vi "decade.vi"(0 "Data In":T5, 2 "Display State In":T3, 3 "Container State":T4) -> (6 "Data Out":T5, 7 "Display State Out":T3, 8 "Action":T2)   [LabVIEW 2017, in "XGaussfitGraph.lvlib" / "XGaussfitGraph.xctl"]
uses:
  XGaussfitGraph.xctl
  Data.ctl
  <vilib>/_xctls/Container State.ctl
  State.ctl
  <vilib>/_xctls/Action.ctl
  Support/Def-UI-Properties.ctl
  <vilib>/_xctls/XControlSupport.lvlib
panel:
  out "Props":T1
  out "Data":dbl[][](graph)
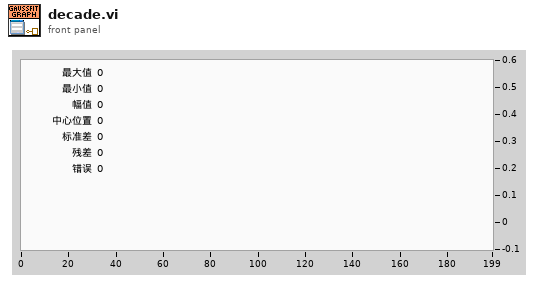
[diagram p1: front panel]
types:
  T1 = typedef "XGaussfitGraph.lvlib/XGaussfitGraph.xctl/Def-UI-Properties.ctl" = cluster{"max value":dbl, "min value":dbl, "amplitude":dbl, "center":dbl, "deviation":dbl, "residue":dbl, "error":i32}
  T2 = typedef "XControlSupport.lvlib/Action.ctl" = cluster{"Data Changed?":bool, "State Changed?":bool, "Action Name":string}
  T3 = typedef "XGaussfitGraph.lvlib/XGaussfitGraph.xctl/State.ctl" = cluster{"Numeric":dbl, "Y.scale":cluster{"auto?":bool, "max":dbl, "min":dbl}}
  T4 = typedef "XControlSupport.lvlib/Container State.ctl" = cluster{"Indicator?":bool, "Run Mode?":bool, " Refnum":refnum<vi>}
  T5 = typedef "XGaussfitGraph.lvlib/XGaussfitGraph.xctl/Data.ctl" = dbl[]
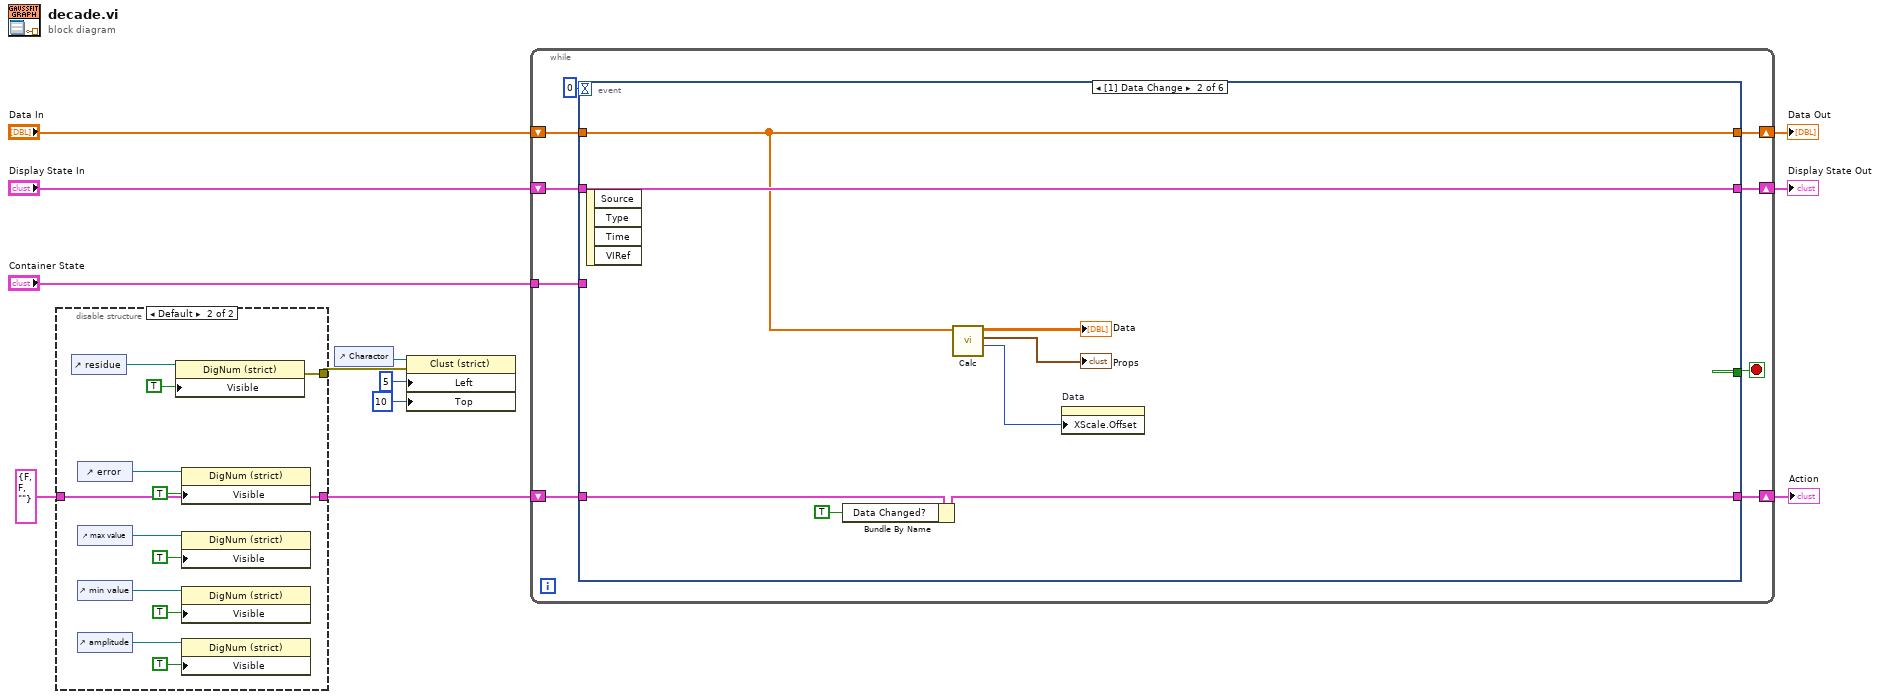
[diagram p0: block diagram]
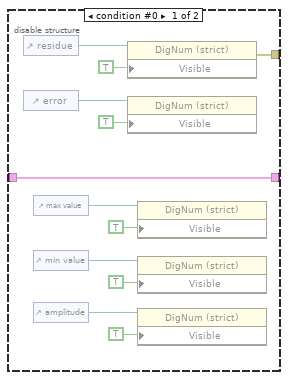
[diagram p2: hidden frame]
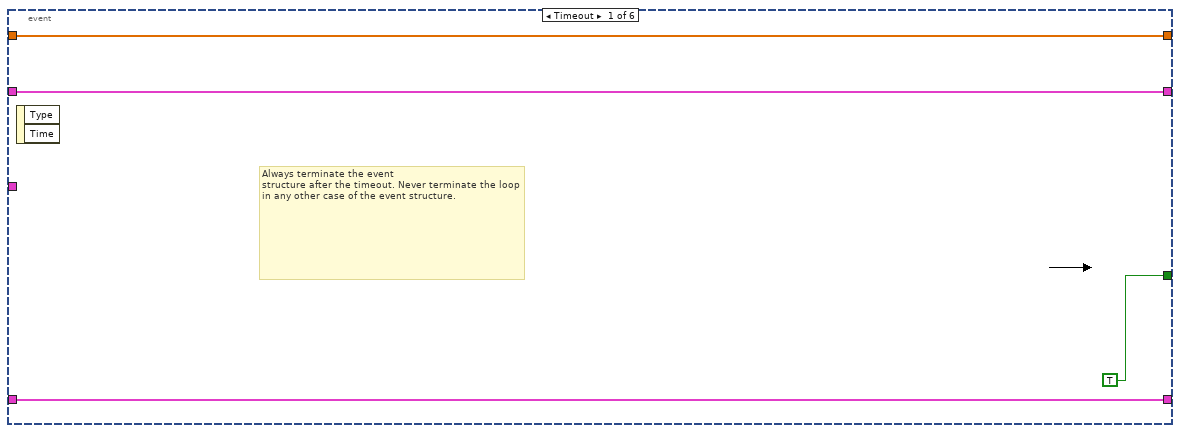
[diagram p3: hidden frame]
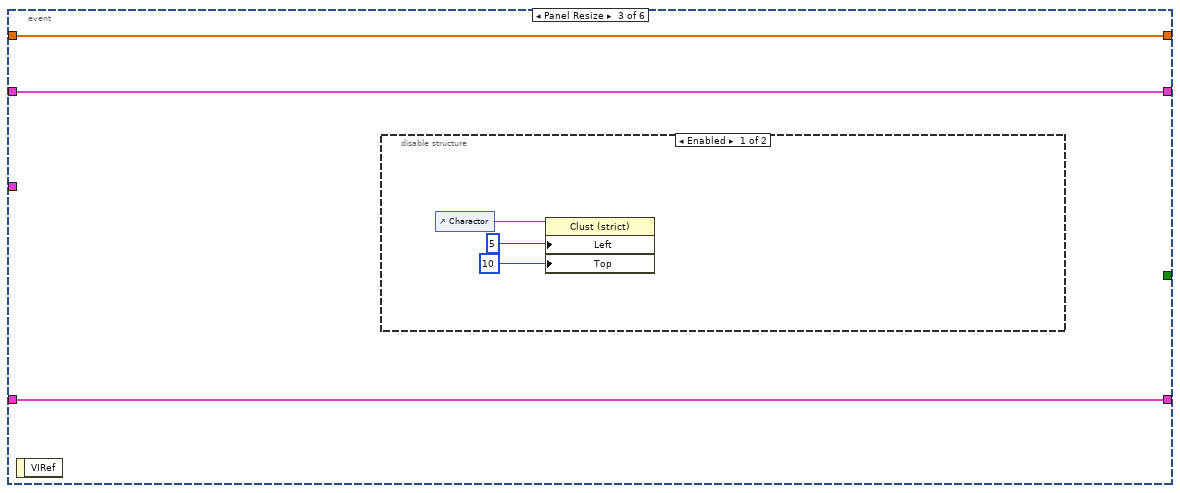
[diagram p4: hidden frame]
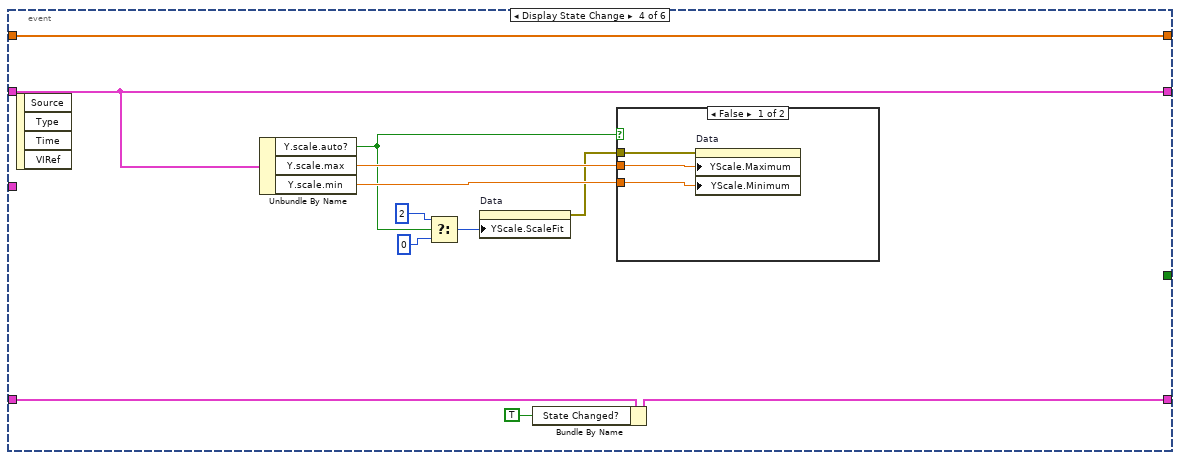
[diagram p6: hidden frame]
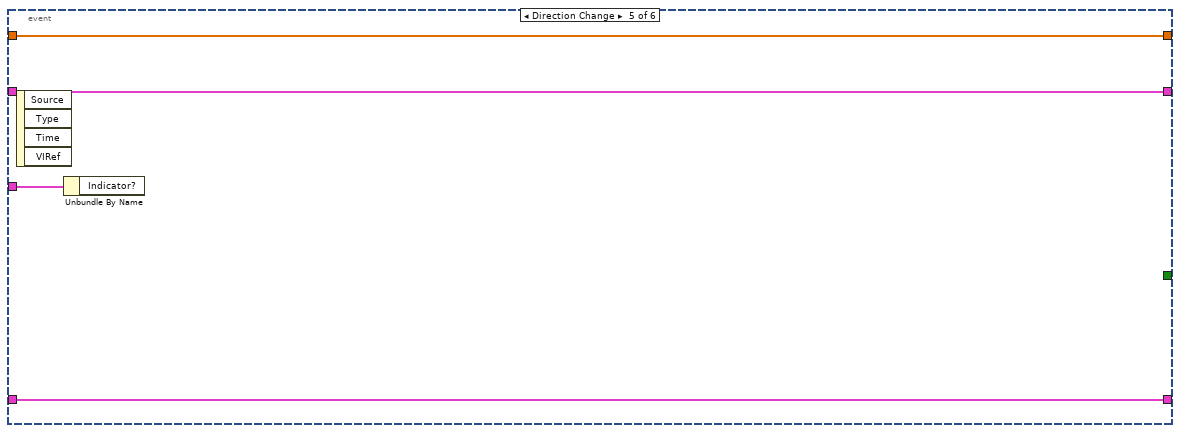
[diagram p8: hidden frame]
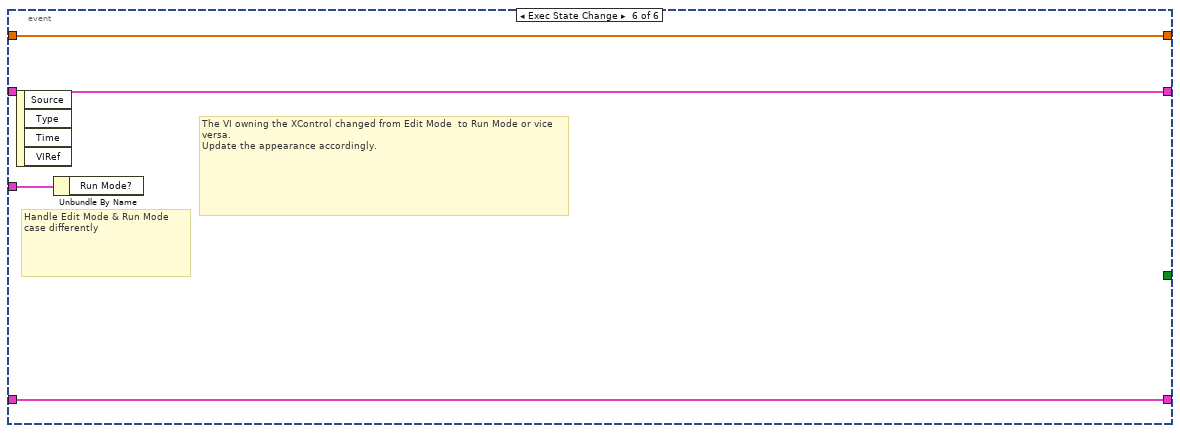
[diagram p9: hidden frame]
diagram:
  n1 = disable-structure shown="Default" {
    disable-tunnel: [w20 w34] -> w6
    disable-tunnel: T2 {"Data Changed?"=FALSE, "State Changed?"=FALSE, "Action Name"=""} ("Action") -> [w20 w34]
    disable-tunnel: [w13 w25] -> w1
    frame condition #0 {
      n2 = control-ref of="residue"() -> (w24:refnum<vi>)
      n3 = control-ref of="error"() -> (w21:refnum<vi>)
      n4 = control-ref of="max value"() -> (w16:refnum<vi>)
      n5 = control-ref of="min value"() -> (w19:refnum<vi>)
      n6 = control-ref of="amplitude"() -> (w14:refnum<vi>)
      n7 = property class="DigNum (strict)"(reference=w24, "Visible"=TRUE) -> (error out=w13:errorcluster)  [unwired: 1 in, 1 out]
      n8 = property class="DigNum (strict)"(reference=w21, "Visible"=TRUE) -> ()  [unwired: 1 in, 2 out]
      n9 = property class="DigNum (strict)"(reference=w16, "Visible"=TRUE) -> ()  [unwired: 1 in, 2 out]
      n10 = property class="DigNum (strict)"(reference=w19, "Visible"=TRUE) -> ()  [unwired: 1 in, 2 out]
      n11 = property class="DigNum (strict)"(reference=w14, "Visible"=TRUE) -> ()  [unwired: 1 in, 2 out]
    }
    frame condition #1 (active) {
      n12 = control-ref of="residue"() -> (w36:refnum<vi>)
      n13 = control-ref of="error"() -> (w32:refnum<vi>)
      n14 = control-ref of="max value"() -> (w28:refnum<vi>)
      n15 = control-ref of="min value"() -> (w31:refnum<vi>)
      n16 = control-ref of="amplitude"() -> (w26:refnum<vi>)
      n17 = property class="DigNum (strict)"(reference=w36, "Visible"=TRUE) -> (error out=w25:errorcluster)  [unwired: 1 in, 1 out]
      n18 = property class="DigNum (strict)"(reference=w32, "Visible"=TRUE) -> ()  [unwired: 1 in, 2 out]
      n19 = property class="DigNum (strict)"(reference=w28, "Visible"=TRUE) -> ()  [unwired: 1 in, 2 out]
      n20 = property class="DigNum (strict)"(reference=w31, "Visible"=TRUE) -> ()  [unwired: 1 in, 2 out]
      n21 = property class="DigNum (strict)"(reference=w26, "Visible"=TRUE) -> ()  [unwired: 1 in, 2 out]
    }
  }
  n22 = control-ref of="Charactor"() -> (w2:refnum<vi>)
  n23 = property class="Clust (strict)"(reference=w2, error in=w1, "Left"=5 ("Position:Left"), "Top"=10 ("Position:Top")) -> ()  [unwired: 2 out]
  n24 = while {
    shift-right: [w44] -> w9
    shift-left: "Display State In" -> [w45]
    tunnel: "Container State" -> [w41]
    shift-right: [w39] -> w12
    shift-left: "Data In" -> [w40]
    shift-right: [w37] -> w7
    shift-left: w6 -> [w38]
    stop <- w43 stop-if-true
    n25 = event shown="[1] Data Change" {
      selector: _ -> [_ _ _ _ _ _]
      dyn-events: _ -> [_ _ _ _ _ _]
      timeout: 0 -> [_ _ _ _ _ _]
      tunnel: w45 -> [w47 w57 w60 w73 w81 w85]
      tunnel: [w47 w57 w60 w73 w81 w85] -> w44
      tunnel: [TRUE _ _ _ _ _] -> w43
      tunnel: w41 -> [_ _ _ _ w82 w86]
      tunnel: w40 -> [w46 w53 w59 w74 w80 w84]
      tunnel: [w46 w53 w59 w74 w80 w84] -> w39
      tunnel: [w48 w55 w58 w65 w79 w83] -> w37
      tunnel: w38 -> [w48 w56 w58 w75 w79 w83]
      event Timeout {
        # "Always terminate the event\nstructure after the timeout. Never terminate the loop in any other case of the event structure."
        n26 = event-data() -> ()  [unwired: 1 in, 2 out]
      }
      event Data Change {
        n27 = event-data() -> ()  [unwired: 1 in, 4 out]
        n28 = Bundle By Name(cluster=w56, "Data Changed?"=TRUE) -> (w55:T2)
        n29 = call "Calc.vi"("Y"=w53) -> ("x-axis Shift"=w50:i32, "properties"=→"Props":T1, "graphs"=→"Data":dbl[][])  [unwired: 7 in, 1 out]
        n30 = property on="Data" class="WFGraph (strict)"("XScale.Offset"=w50) -> ()  [unwired: 2 in, 2 out]
      }
      event Panel Resize {
        n31 = event-data() -> ()  [unwired: 1 in, 1 out]
        n32 = disable-structure shown="Enabled" {
          frame Enabled {
            n33 = control-ref of="Charactor"() -> (w63:refnum<vi>)
            n34 = property class="Clust (strict)"(reference=w63, "Left"=5 ("Position:Left"), "Top"=10 ("Position:Top")) -> ()  [unwired: 1 in, 2 out]
          }
          frame Disabled {
          }
        }
      }
      event Display State Change {
        n35 = event-data() -> ()  [unwired: 1 in, 4 out]
        n36 = Unbundle By Name(w73) -> ("Y.scale.auto?"=w66:bool, "Y.scale.max"=w72:dbl, "Y.scale.min"=w71:dbl)
        n37 = Select(t=u8 2 ("Y Scale.Scale Fit"), s=w66, f=u8 0 ("Y Scale.Scale Fit")) -> (s? t:f=w70:u8)
        n38 = property on="Data" class="WFGraph (strict)"("YScale.ScaleFit"=w70) -> (error out=w67:errorcluster)  [unwired: 2 in, 1 out]
        n39 = Bundle By Name(cluster=w75, "State Changed?"=TRUE) -> (w65:T2)
        n40 = case shown="False" w66 {
          tunnel: w72 -> [w78 _]
          tunnel: w71 -> [w77 _]
          tunnel: w67 -> [w76 _]
          frame False {
            n41 = property on="Data" class="WFGraph (strict)"(error in=w76, "YScale.Maximum"=w78, "YScale.Minimum"=w77) -> ()  [unwired: 1 in, 2 out]
          }
          frame True {
          }
        }
      }
      event Direction Change {
        n42 = event-data() -> ()  [unwired: 1 in, 4 out]
        n43 = Unbundle By Name(w82) -> ()  [unwired: 1 out]
      }
      event Exec State Change {
        # "The VI owning the XControl changed from Edit Mode  to Run Mode or vice versa.\nUpdate the appearance accordingly."
        # "Handle Edit Mode & Run Mode\ncase differently"
        n44 = event-data() -> ()  [unwired: 1 in, 4 out]
        n45 = Unbundle By Name(w86) -> ()  [unwired: 1 out]
      }
    }
  }
  "Display State Out" <- w9
  "Data Out" <- w12
  "Action" <- w7
